vi "RT Driver VI.vi"(7 "Operation":T1, 11 "Device Reference in":T2 format="%.0x") -> (0 "Error Code":i32)   [LabVIEW 2020, in "Ballard MIL-1553 Engine.lvlib"]
uses:
  Ballard MIL-1553 Engine.lvlib
  <vilib>/NI VeriStand/Custom Device API/Custom Device Item Ref.ctl
  <vilib>/NI VeriStand/Custom Device API/Hardware Interface Driver VI Operation.ctl
  RT Driver/Controls/RT StateVariables.ctl
  <vilib>/NI/NIVS Inline Async API/_VS Inline Async API/VS Inline Async API/VS Inline Async API.lvclass
  RT Driver/Controls/Card Parameters.ctl
  Shared/Controls and Global/Initialization Method.ctl
  <vilib>/NI VeriStand/Custom Device API/Data Reference.ctl
  RT Driver/Controls/RT Inline Data_Data Description_Channel.ctl
  RT Driver/Controls/RT Inline Frame Descriptor.ctl
  RT Driver/Controls/RT Inline Frame Descriptor_BC.ctl
  <vilib>/NI VeriStand/Custom Device API/Block Data Reference.ctl
  Shared/EncodeDecode/_typedefs/parameter_config_type.ctl
  Shared/EncodeDecode/_typedefs/parameter_config_type_type.ctl
  Shared/EncodeDecode/_typedefs/parameter_config_encoding_type.ctl
  RT Driver/Controls/RT Inline Frame Descriptor_RT.ctl
  Shared/Controls and Global/RT CWD2.ctl
  Shared/Controls and Global/RT CWD1.ctl
  Shared/Controls and Global/RT messageType.ctl
  <vilib>/NI/NIVS Inline Async API/_VS Inline Async API/VS Inline Async API/VS Inline Async API.lvclass/VS Inline Async API.ctl
  <vilib>/NI/NIVS Inline Async API/_Data Access Engine/Data Access Engine/Data Access Engine.lvclass/Data Access Engine.ctl
  <vilib>/NI/NIVS Inline Async API/_Data Access Engine/Access Type Classes/Write/Write.lvclass/Write.ctl
  <vilib>/NI/NIVS Inline Async API/_Data Access Engine/Access Type Classes/ReadWrite/ReadWrite.lvclass/ReadWrite.ctl
  RT Driver/Controls/Inline_Status_Channels.ctl
  <vilib>/NI/NIVS Inline Async API/_Data Access Engine/Access Type Classes/Read/Read.lvclass/Read.ctl
  <vilib>/NI/NIVS Inline Async API/_Data Access Engine/Data Access Engine/Methods/Data.Engine.Read Data from HW.vi
  <vilib>/NI/NIVS Inline Async API/_VS Inline Async API/Error Handling Process/SubVIs/Error.GetError.vi
  <vilib>/NI/NIVS Inline Async API/_Data Access Engine/Data Access Engine/Methods/Data.Engine.Write Data to HW.vi
  <vilib>/NI/NIVS Inline Async API/_Data Access Engine/Access Type Classes/ReadWrite/ReadWrite.EngineData.vi
  <vilib>/NI/NIVS Inline Async API/_Data Access Engine/Access Type Classes/Write/Write.EngineData.vi
  <vilib>/NI/NIVS Inline Async API/_Data Access Engine/Access Type Classes/Read/Read.EngineData.vi
  <vilib>/NI VeriStand/Custom Device API/NI VeriStand - Get Channel Value by Data Reference.vi
  <vilib>/NI VeriStand/Custom Device API/NI VeriStand - Set Channel Value by Data Reference.vi
  <vilib>/NI VeriStand/Custom Device API/NI VeriStand - Get Channel Values by Block Data Reference.vi
  <vilib>/NI VeriStand/Custom Device API/Global Data Refs.vi
  Shared/Ballard 1553 Shared.lvlib
  <vilib>/NI VeriStand/Custom Device API/Custom Device API.lvlib
panel:
  out "Write time uS":u32
  out "Read time uS":u32
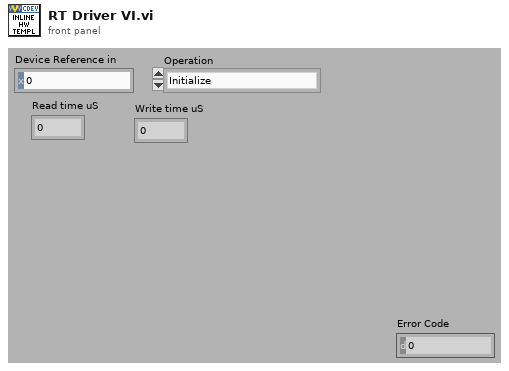
[diagram p1: front panel]
types:
  T1 = typedef "Custom Device API.lvlib/Hardware Interface Driver VI Operation.ctl" = enum16{"Initialize", "Start", "Read Data from HW", "Write Data to HW", "Close"}
  T2 = typedef "Custom Device API.lvlib/Custom Device Item Ref.ctl" = u64
  T3 = typedef "Custom Device API.lvlib/Custom Device Item Info.ctl" = cluster{"Name":string, "Is Channel":bool, "GUID":string, "Is Waveform":bool}
  T4 = typedef "Ballard MIL-1553 Engine.lvlib/RT StateVariables.ctl" = cluster{"Async":refnum<class "VS Inline Async API.lvclass">, "Card Parameters (out)":T5, "Inline Status Channels Refs":T7[], "RT Inline Data_Data Description_Channels":T8[]}
  T5 = typedef "Ballard MIL-1553 Engine.lvlib/Card Parameters.ctl" = cluster{"card number":i32, "core number":i32, "core handle":u64, "core reader handle":u64, "channel handles[]":u64[], "Initialization Method":T6, "PXI slot number":i32}
  T6 = typedef "Ballard 1553 Shared.lvlib/Initialization Method.ctl" = enum16{"PXI Slot Number", "Card Number"}
  T7 = typedef "Custom Device API.lvlib/Data Reference.ctl" = i32
  T8 = typedef "Ballard MIL-1553 Engine.lvlib/RT Inline Data_Data Description_Channel.ctl" = cluster{"hardwareChannel":u16, "First Index for RT2RT Frames":i32, "Frame Drescriptors":T9[]}
  T9 = typedef "Ballard MIL-1553 Engine.lvlib/RT Inline Frame Descriptor.ctl" = cluster{"BC":T10, "RT":T15, "Initialized?":bool, "RT to RT?":bool, "CWD2":T16, "CWD1":T17, "messageType":T18, "Name":string}
  T10 = typedef "Ballard MIL-1553 Engine.lvlib/RT Inline Frame Descriptor_BC.ctl" = cluster{"Timestamp?":bool, "Timestamp Channel Data Reference":T7, "Data Words?":bool, "param block data refs":T11[], "Sw1?":bool, "Sw2?":bool, "Status Channel Refs":T2[], "ParamConfig":T12[], "word_count":u8}
  T11 = typedef "Custom Device API.lvlib/Block Data Reference.ctl" = cluster{"Data Reference":T7, "Offset":u64, "Length":u64}
  T12 = typedef "parameter_config_type.ctl" = cluster{"Name":string, "Type":T13, "Units":string, "Nword":i32, "StartBit":i32, "Size":i32, "LSB_Value":dbl, "Offset":i32, "Encoding":T14}
  T13 = typedef "parameter_config_type_type.ctl" = enum16{"Opaque", "Enum", "Float", "Integer", "Bcd", "Bool"}
  T14 = typedef "parameter_config_encoding_type.ctl" = enum16{"None", "2-complement", "Unsigned"}
  T15 = typedef "Ballard MIL-1553 Engine.lvlib/RT Inline Frame Descriptor_RT.ctl" = cluster{"Timestamp?":bool, "Timestamp Channel Data Reference":T7, "Data Words?":bool, "Words Block Data Refs":T11[], "Status Channel Ref?":bool, "Status Channel Ref":T2, "ParamConfig":T12[], "word_count":u8}
  T16 = typedef "Ballard 1553 Shared.lvlib/RT CWD2.ctl" = cluster{"TA (RT)":i8, "SA":i8, "Words (WC)":i8}
  T17 = typedef "Ballard 1553 Shared.lvlib/RT CWD1.ctl" = cluster{"TA (RT)":i8, "SA":i8, "Mode Code":i8, "Words Count":i8}
  T18 = typedef "Ballard 1553 Shared.lvlib/RT messageType.ctl" = enum16{"BC to RT", "RT to BC", "RT to RT", "MC (Rx)", "MC (Tx)"}
  T19 = typedef "Ballard MIL-1553 Engine.lvlib/Inline_Status_Channels.ctl" = enum16{"Error Code", "Inline Read Time (us)", "Inline Write Time (us)", "Unconfigured Frames Counter", "Monitor - Error Counter", "General Protocol Error Counter", "Wrong Sync Error Counter", "Improper Number of Data Words Error", "Manchester Error Counter", "Parity Error Counter", "Word Error Counter"}
  T20 = typedef "Ballard MIL-1553 Engine.lvlib/RT Async Data.ctl" = cluster{"Map (BC to RT)":T21[], "Raw Values (BC to RT)":T23, "param map (BC to RT)":T25, "Map (RT to ..)":T26[], "Raw Values (RT to ..)":T23, "param map (RT to BC)":T25, "Map (RTs Status)":T27[], "Raw Values (RTs Status)":T23, "Map (Bc Command Channels)":T28[], "MAP (BC Acyclic Messages Trigger)":T29[], "Map (RT Command Channels)":T30[], "Map (MC Rx)":T21[], "Raw Values (MC Rx)":T23, "param map (MC Rx)":T25, "Raw Values (MC Tx)":T23, "Map (MC Tx)":T26[], "param map (MC Tx)":T25}
  T21 = typedef "Ballard MIL-1553 Engine.lvlib/RT Async_Map BC2RT.ctl" = cluster{"Channel Index":i32, "ID":i32, "Channel Data Reference":T7, "Word Index":i32, "Message Handle":u64, "Type":T22, "Word Count":i32, "First Element Index":i32}
  T22 = typedef "Ballard MIL-1553 Engine.lvlib/RT Async_Map_Type.ctl" = enum16{"Word (BC to RT)", "Word (MC (Rx))", "Acyclic Message Trigger", "Word (RT to ..)", "Word (RT to RT)", "Word (MC (Tx))", "RT Status", "BC Commands", "RT Commands"}
  T23 = typedef "Ballard MIL-1553 Engine.lvlib/RT Async_Raw Values.ctl" = cluster{"Association":T24[], "Raw Values Array":u16[]}
  T24 = typedef "Ballard MIL-1553 Engine.lvlib/RT Async_Raw Values to Messages Index_Association.ctl" = cluster{"Message Index":i32, "Raw Value Index":i32}
  T25 = typedef "Ballard MIL-1553 Engine.lvlib/Asynchronous - Parameter map_type.ctl" = cluster{"ParamConfig":T12[], "word_count":u8[], "param_count":u8[]}
  T26 = typedef "Ballard MIL-1553 Engine.lvlib/RT Async_Map RT2BC.ctl" = cluster{"Channel Index":i32, "ID":i32, "Word Data Reference":T7, "First element Index":i32, "rt Transfer Handle":u64, "Type":T22, "Word Count":i32}
  T27 = typedef "Ballard MIL-1553 Engine.lvlib/RT Async_Map RTs Status.ctl" = cluster{"Channel Index":i32, "ID":i32, "rt Transfer Handle":u64, "Type":T22}
  T28 = typedef "Ballard MIL-1553 Engine.lvlib/RT Async_Map BC Command Channels.ctl" = cluster{"Channel Index":i32, "ID":i32, "BC Handle":u64, "Type":T22, "BC Command Channel Ref":T2, "Command Type":enum16{"Start Command", "Stop Command"}}
  T29 = typedef "Ballard MIL-1553 Engine.lvlib/RT Async_Map BC Acyclic Messages Trigger.ctl" = cluster{"Channel Index":i32, "BC Handle":u64, "Type":T22, "Acyclic Message Trigger Channel Ref":T2, "Message Name":string}
  T30 = typedef "Ballard MIL-1553 Engine.lvlib/RT Async_Map RT Command Channels.ctl" = cluster{"Channel Index":i32, "ID":i32, "RT Handle":u64, "Type":T22, "RT Command Channel Ref":T2, "Command Type":enum16{"Start Command", "Stop Command"}}
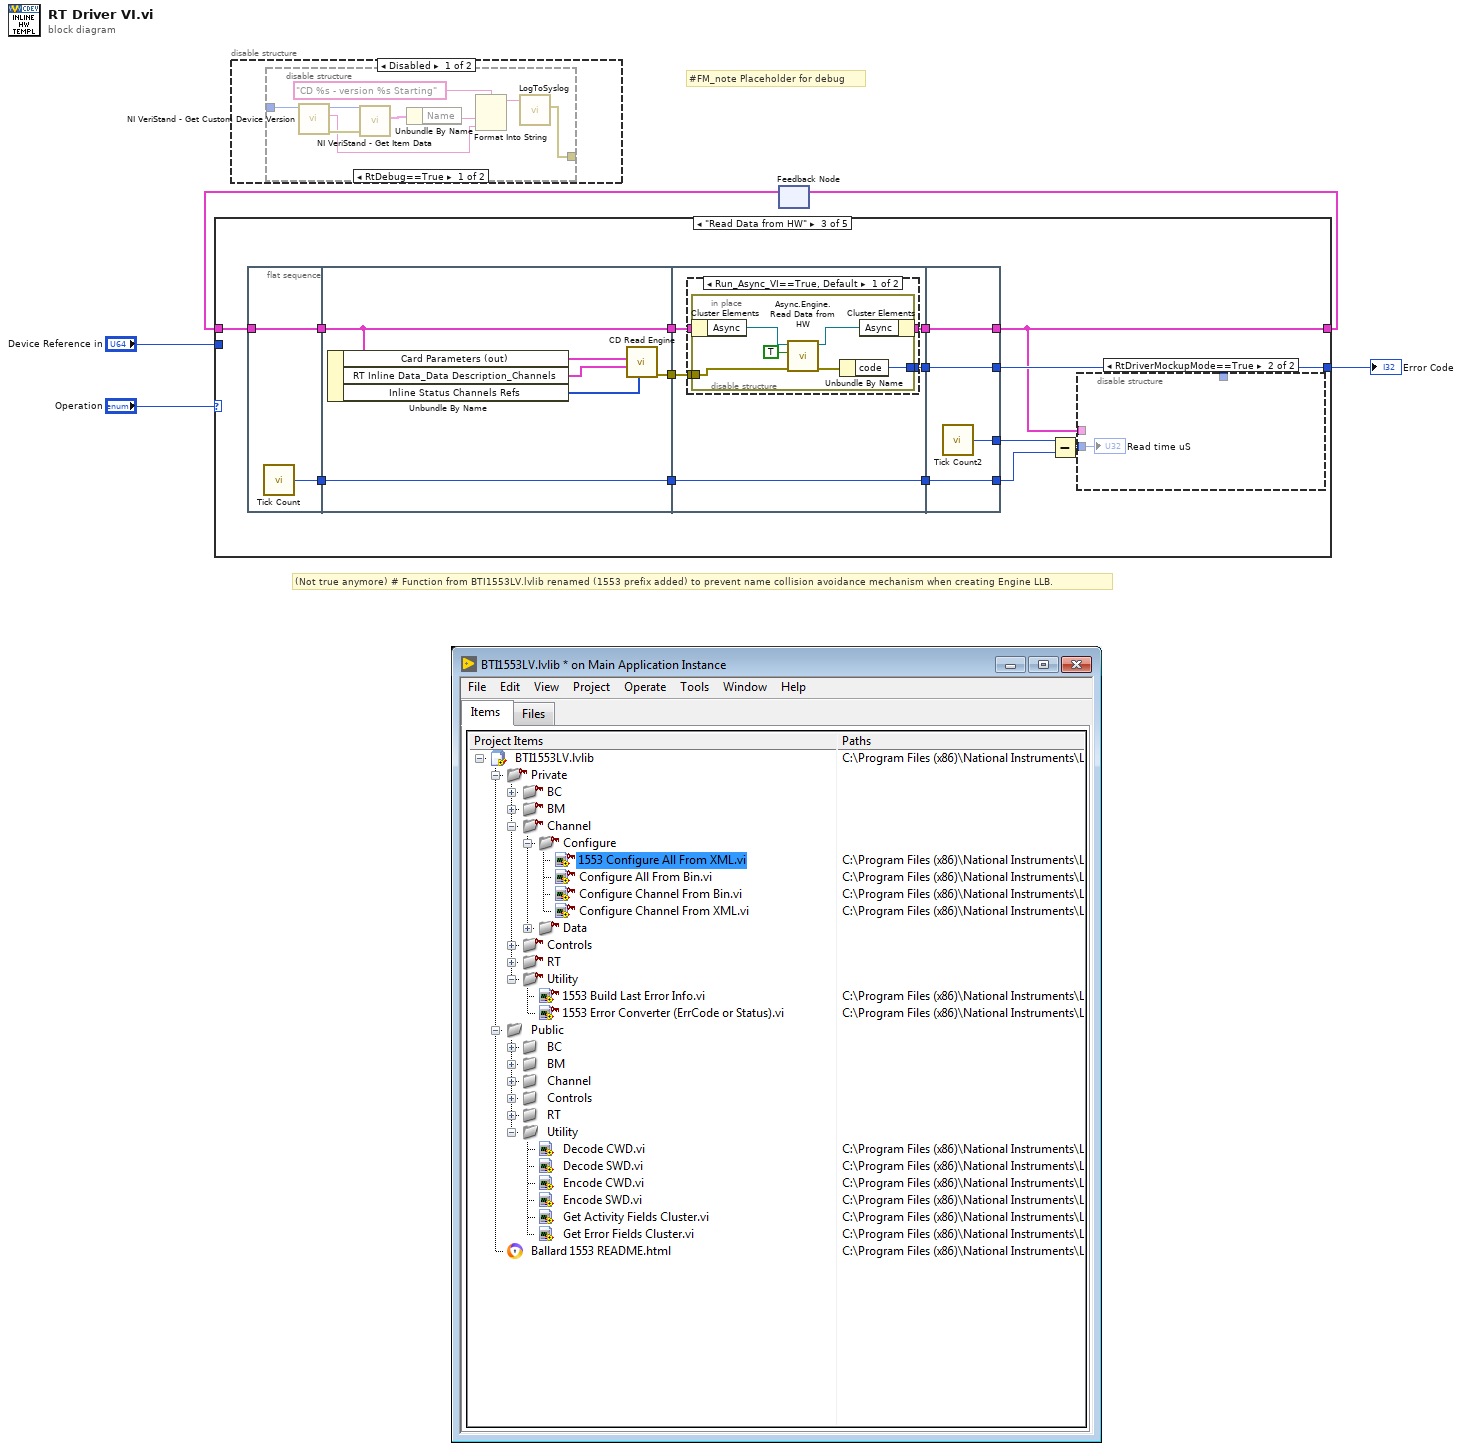
[diagram p0: block diagram]
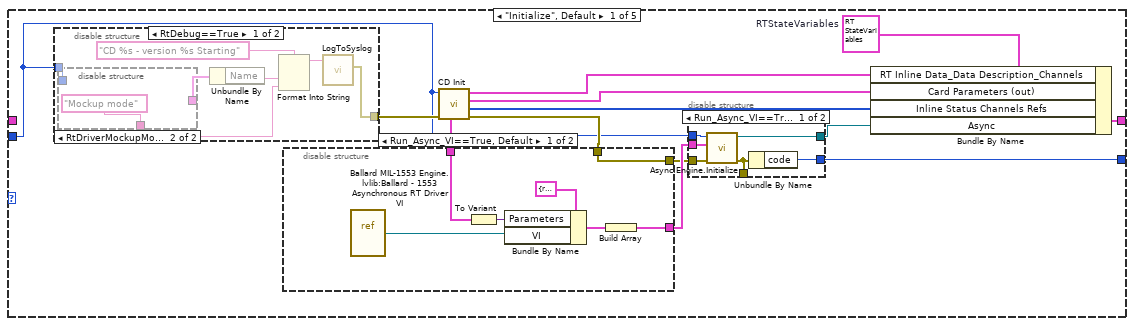
[diagram p4: hidden frame]
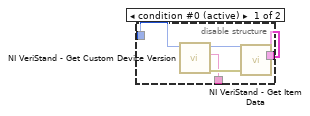
[diagram p5: hidden frame]
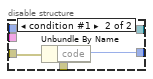
[diagram p8: hidden frame]
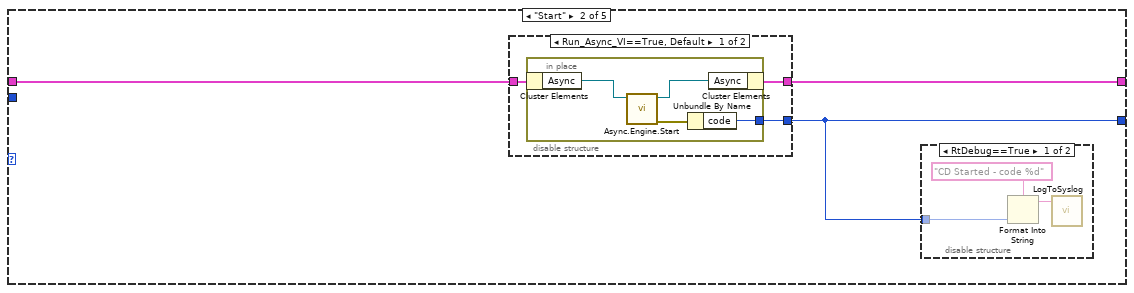
[diagram p9: hidden frame]
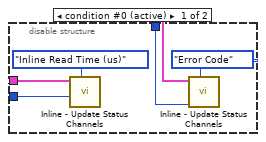
[diagram p12: hidden frame]
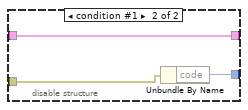
[diagram p13: hidden frame]
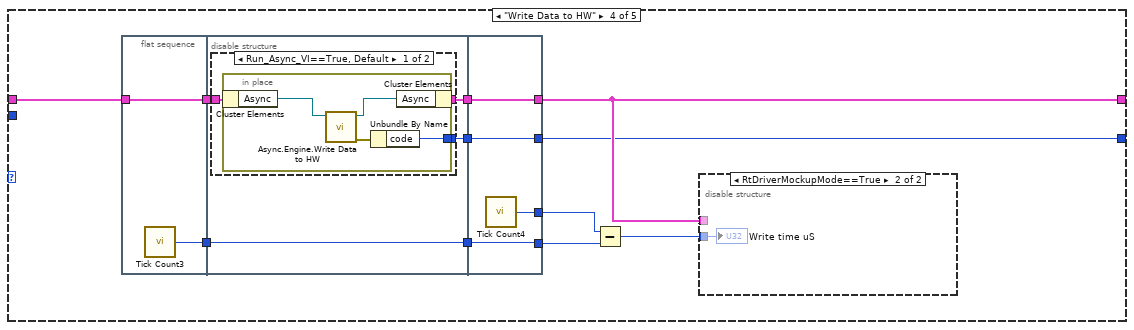
[diagram p14: hidden frame]
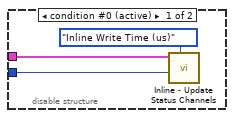
[diagram p15: hidden frame]
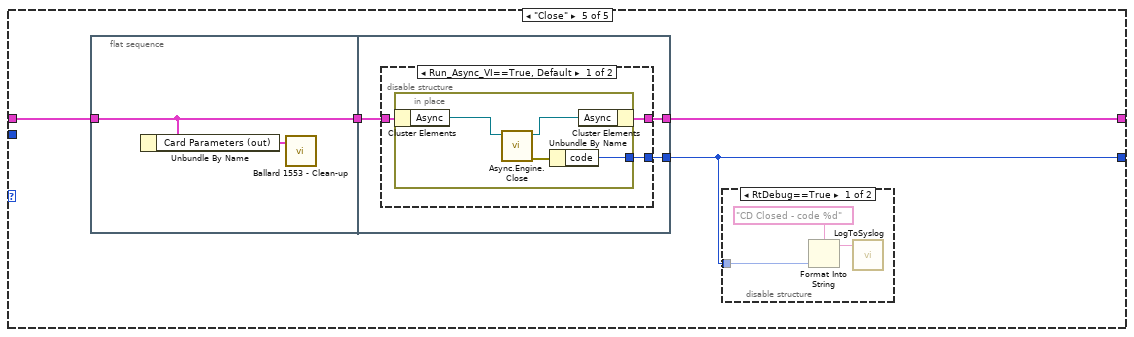
[diagram p17: hidden frame]
diagram:
  # "#FM_note Placeholder for debug"
  # "(Not true anymore) # Function from BTI1553LV.lvlib renamed (1553 prefix added) to prevent name collision avoidance mechanism when creating Engine LLB."
  n1 = disable-structure shown="Disabled" {
    frame Disabled {
      n2 = disable-structure shown="RtDebug==True" {
        disable-tunnel: _ -> [w14 _]
        disable-tunnel: [w8 _] -> _
        frame condition #0 {
          n3 = call <vilib>:"NI VeriStand - Get Custom Device Version.vi"("Device Ref in"=w14) -> ("error out"=w12:errorcluster, "Value"=w6:string, "Device Ref out"=w13:T2)  [unwired: 8 in]
          n4 = call <vilib>:"NI VeriStand - Get Item Data.vi"("error in (no error)"=w12, "Item Ref in"=w13) -> ("Item Info"=w11:T3)  [unwired: 9 out]
          n5 = Unbundle By Name(w11) -> ("Name"=w7:string)
          n6 = Format Into String(format string="CD %s - version %s Starting", w7, w6) -> (resulting string=w10:string)  [unwired: 2 in, 1 out]
          n7 = call "LogToSyslog.vi"("message"=w10) -> ("error out"=w8:errorcluster)  [unwired: 9 in, 1 out]
        }
        frame condition #1 (active) {
        }
      }
    }
    frame Enabled {
    }
  }
  n8 = feedback #1() -> (w4:T4)  [unwired: 1 out]
  n9 = case shown="\"Read Data from HW\"" "Operation" {
    tunnel: [w26 w59 w77 w122 w156] -> w5
    tunnel: w4 -> [_ w58 w84 w131 w157]
    tunnel: "Device Reference in" -> [w15 _ _ _ _]
    tunnel: [w18 w57 w79 w121 w154] -> w1
    frame "Initialize", Default {
      w25 = T4 {"Async"=refnum, "Card Parameters (out)"={"card number"=0, "core number"=0, "core handle"=0, "core reader handle"=0, "channel handles[]"=[], "Initialization Method"=enum."PXI Slot Number", "PXI slot number"=0}, "Inline Status Channels Refs"=[], "RT Inline Data_Data Description_Channels"=[]}  # RTStateVariables
      n10 = disable-structure shown="RtDebug==True" {
        disable-tunnel: w15 -> [w34 _]
        disable-tunnel: [w30 _] -> w16
        frame condition #0 {
          n11 = disable-structure shown="RtDriverMockupMode==True" {
            disable-tunnel: w34 -> [w39 _]
            disable-tunnel: [w36 _] -> w33
            disable-tunnel: [w35 "Mockup mode" ("Value")] -> w28
            frame condition #0 (active) {
              n12 = call <vilib>:"NI VeriStand - Get Custom Device Version.vi"("Device Ref in"=w39) -> ("error out"=w37:errorcluster, "Value"=w35:string, "Device Ref out"=w38:T2)  [unwired: 8 in]
              n13 = call <vilib>:"NI VeriStand - Get Item Data.vi"("error in (no error)"=w37, "Item Ref in"=w38) -> ("Item Info"=w36:T3)  [unwired: 9 out]
            }
            frame condition #1 {
            }
          }
          n14 = Unbundle By Name(w33) -> ("Name"=w29:string)
          n15 = Format Into String(format string="CD %s - version %s Starting", w29, w28) -> (resulting string=w32:string)  [unwired: 2 in, 1 out]
          n16 = call "LogToSyslog.vi"("message"=w32) -> ("error out"=w30:errorcluster)  [unwired: 9 in, 1 out]
        }
        frame condition #1 (active) {
        }
      }
      n17 = call "CD Init.vi"("Error (in)"=w16, "Device Reference"=w15) -> ("Error (out)"=w19:errorcluster, "Inline Status Channels Refs"=w21:T7[], "Card Parameters (out)"=w22:T5, "RT Inline Data_Data Description_Channels"=w23:T8[], "RT Async Data"=w20:T20)  [unwired: 5 in]
      n18 = disable-structure shown="Run_Async_VI==True, Default" {
        disable-tunnel: [w45 _] -> w24
        disable-tunnel: w20 -> [w43 _]
        disable-tunnel: w19 -> [w42 w48]
        disable-tunnel: [w42 w48] -> w17
        frame condition #0 (active) {
          n19 = vi-ref "Ballard MIL-1553 Engine.lvlib:Ballard - 1553 Asynchronous RT Driver VI.vi"() -> (w41:refnum<vi>)
          n20 = To Variant(anything=w43) -> (Variant=w44:variant)
          n21 = Bundle By Name(cluster=cluster{"VI":refnum<vi>, "Parameters":variant} {"VI"=refnum, "Parameters"=variant} ("Process"), "Parameters"=w44, "VI"=w41) -> (w46:cluster{"VI":refnum<vi>, "Parameters":variant})
          n22 = Build Array(w46) -> (w45:cluster{"VI":refnum<vi>, "Parameters":variant}[])
        }
        frame condition #1 {
        }
      }
      n23 = disable-structure shown="Run_Async_VI==True, Default" {
        disable-tunnel: [w54 w55] -> w18
        disable-tunnel: [w53 _] -> w27
        disable-tunnel: w24 -> [w52 _]
        disable-tunnel: w17 -> [w51 w56]
        disable-tunnel: [w50 _] -> _
        disable-tunnel: w15 -> [w49 _]
        frame condition #0 (active) {
          n24 = call <vilib>:"Async.Engine.Initialize.vi"("error in (no error)"=w51, "Processes"=w52, "Custom Device Ref"=w49) -> ("error out"=w50:errorcluster, "Async"=w53:refnum<class "VS Inline Async API.lvclass">)  [unwired: 7 in]
          n25 = Unbundle By Name(w50) -> ("code"=w54:i32)
        }
        frame condition #1 {
          n26 = Unbundle By Name(w56) -> ("code"=w55:i32)
        }
      }
      n27 = Bundle By Name(cluster=w25, "RT Inline Data_Data Description_Channels"=w23, "Card Parameters (out)"=w22, "Inline Status Channels Refs"=w21, "Async"=w27) -> (w26:T4)
    }
    frame "Start" {
      n28 = disable-structure shown="Run_Async_VI==True, Default" {
        disable-tunnel: w58 -> [w65 w70]
        disable-tunnel: [w64 w70] -> w59
        disable-tunnel: [w63 _] -> w57
        frame condition #0 (active) {
          n29 = in-place {
            in-place-border: [w66] -> w63
            n30 = in-place-cluster #2(w65) -> ("Async"=w69:refnum<class "VS Inline Async API.lvclass">)
            n31 = call <vilib>:"Async.Engine.Start.vi"("VS Inline Async API in"=w69) -> ("error out"=w67:errorcluster, "VS Inline Async API out"=w68:refnum<class "VS Inline Async API.lvclass">)  [unwired: 9 in]
            n32 = Unbundle By Name(w67) -> ("code"=w66:i32)
            n33 = in-place-cluster #2("Async"=w68) -> (w64:T4)
          }
        }
        frame condition #1 {
        }
      }
      n34 = disable-structure shown="RtDebug==True" {
        disable-tunnel: w57 -> [w60 _]
        frame condition #0 {
          n35 = Format Into String(format string="CD Started - code %d", w60) -> (resulting string=w62:string)  [unwired: 2 in, 1 out]
          n36 = call "LogToSyslog.vi"("message"=w62) -> ()  [unwired: 9 in, 2 out]
        }
        frame condition #1 (active) {
        }
      }
    }
    frame "Read Data from HW" {
      n37 = flat-sequence {
        tunnel: w84 -> [w92]
        tunnel: [w92] -> w83
        tunnel: [w91] -> w82
        tunnel: [w97] -> w76
        tunnel: [w98] -> w74
        tunnel: w82 -> [w98]
        tunnel: w83 -> [w97]
        tunnel: [w96] -> w71
        tunnel: w76 -> [w102]
        tunnel: [w101] -> w75
        tunnel: w74 -> [w103]
        tunnel: [w103] -> w73
        tunnel: [w99] -> w72
        tunnel: w71 -> [w100]
        tunnel: [w119] -> w77
        tunnel: [w120] -> w79
        tunnel: w75 -> [w119]
        tunnel: [w118] -> w81
        tunnel: w73 -> [w117]
        tunnel: [w117] -> w80
        tunnel: w72 -> [w120]
        frame #0 {
          n38 = call "Tick Count"() -> ("Tick Count(uSec)"=w91:u32)
        }
        frame #1 {
          n39 = Unbundle By Name(w97) -> ("Card Parameters (out)"=w95:T5, "RT Inline Data_Data Description_Channels"=w93:T8[], "Inline Status Channels Refs"=w94:T7[])
          n40 = call "CD Read Engine.vi"("Inline Status Channels Refs"=w94, "RT Inline Data_Data Description_Channels"=w93, "Card Parameters (in)"=w95) -> ("Error (out)"=w96:errorcluster)  [unwired: 7 in]
        }
        frame #2 {
          n41 = disable-structure shown="Run_Async_VI==True, Default" {
            disable-tunnel: [w107 w114] -> w99
            disable-tunnel: w102 -> [w106 w116]
            disable-tunnel: [w105 w116] -> w101
            disable-tunnel: w100 -> [w104 w115]
            frame condition #0 (active) {
              n42 = in-place {
                in-place-border: [w111] -> w107
                in-place-border: w104 -> [w108]
                n43 = in-place-cluster #3(w106) -> ("Async"=w113:refnum<class "VS Inline Async API.lvclass">)
                n44 = call <vilib>:"Async.Engine.Read Data from HW.vi"("error in"=w108, "Report Error to Inline?"=TRUE, "Async in"=w113) -> ("error out"=w110:errorcluster, "Async out"=w112:refnum<class "VS Inline Async API.lvclass">)  [unwired: 7 in]
                n45 = Unbundle By Name(w110) -> ("code"=w111:i32)
                n46 = in-place-cluster #3("Async"=w112) -> (w105:T4)
              }
            }
            frame condition #1 {
              n47 = Unbundle By Name(w115) -> ("code"=w114:i32)
            }
          }
        }
        frame #3 {
          n48 = call "Tick Count2"() -> ("Tick Count(uSec)"=w118:u32)
        }
      }
      n49 = Subtract(x=w81, y=w80) -> (x-y=w78:u32)
      n50 = disable-structure shown="RtDriverMockupMode==True" {
        disable-tunnel: w79 -> [w89 _]
        disable-tunnel: w78 -> [w87 w90]
        disable-tunnel: w77 -> [w86 _]
        frame condition #0 (active) {
          n51 = call "Inline - Update Status Channels.vi"("Status Channel"=Inline_Status_Channels."Inline Read Time (us)", "Time (us)"=w87, "RTStateVariables"=w86) -> ()  [unwired: 9 in]
          n52 = call "Inline - Update Status Channels.vi"("Status Channel"=Inline_Status_Channels."Error Code", "Error Code"=w89, "RTStateVariables"=w86) -> ()  [unwired: 9 in]
        }
        frame condition #1 {
          "Read time uS" <- w90
        }
      }
    }
    frame "Write Data to HW" {
      n53 = flat-sequence {
        tunnel: w131 -> [w137]
        tunnel: [w137] -> w130
        tunnel: [w136] -> w127
        tunnel: w130 -> [w138]
        tunnel: [w141] -> w129
        tunnel: [w140] -> w128
        tunnel: w127 -> [w139]
        tunnel: [w139] -> w126
        tunnel: [w152] -> w122
        tunnel: [w153] -> w121
        tunnel: w129 -> [w153]
        tunnel: w128 -> [w152]
        tunnel: [w151] -> w124
        tunnel: w126 -> [w150]
        tunnel: [w150] -> w125
        frame #0 {
          n54 = call "Tick Count3"() -> ("Tick Count(uSec)"=w136:u32)
        }
        frame #1 {
          n55 = disable-structure shown="Run_Async_VI==True, Default" {
            disable-tunnel: [w144 _] -> w141
            disable-tunnel: w138 -> [w143 w149]
            disable-tunnel: [w142 w149] -> w140
            frame condition #0 (active) {
              n56 = in-place {
                in-place-border: [w148] -> w144
                n57 = in-place-cluster #4(w143) -> ("Async"=w146:refnum<class "VS Inline Async API.lvclass">)
                n58 = call <vilib>:"Async.Engine.Write Data to HW.vi"("VS Inline Async API in"=w146) -> ("error out"=w147:errorcluster, "VS Inline Async API out"=w145:refnum<class "VS Inline Async API.lvclass">)  [unwired: 9 in]
                n59 = Unbundle By Name(w147) -> ("code"=w148:i32)
                n60 = in-place-cluster #4("Async"=w145) -> (w142:T4)
              }
            }
            frame condition #1 {
            }
          }
        }
        frame #2 {
          n61 = call "Tick Count4"() -> ("Tick Count(uSec)"=w151:u32)
        }
      }
      n62 = Subtract(x=w124, y=w125) -> (x-y=w123:u32)
      n63 = disable-structure shown="RtDriverMockupMode==True" {
        disable-tunnel: w123 -> [w134 w135]
        disable-tunnel: w122 -> [w133 _]
        frame condition #0 (active) {
          n64 = call "Inline - Update Status Channels.vi"("Status Channel"=Inline_Status_Channels."Inline Write Time (us)", "Time (us)"=w134, "RTStateVariables"=w133) -> ()  [unwired: 9 in]
        }
        frame condition #1 {
          "Write time uS" <- w135
        }
      }
    }
    frame "Close" {
      n65 = flat-sequence {
        tunnel: w157 -> [w162]
        tunnel: [w162] -> w155
        tunnel: [w164] -> w156
        tunnel: [w163] -> w154
        tunnel: w155 -> [w165]
        frame #0 {
          n66 = Unbundle By Name(w162) -> ("Card Parameters (out)"=w161:T5)
          n67 = call "Ballard 1553 - Clean-up.vi"("Card Parameters"=w161) -> ()  [unwired: 10 in, 1 out]
        }
        frame #1 {
          n68 = disable-structure shown="Run_Async_VI==True, Default" {
            disable-tunnel: w165 -> [w168 w173]
            disable-tunnel: [w167 w173] -> w164
            disable-tunnel: [w166 _] -> w163
            frame condition #0 (active) {
              n69 = in-place {
                in-place-border: [w170] -> w166
                n70 = in-place-cluster #5(w168) -> ("Async"=w172:refnum<class "VS Inline Async API.lvclass">)
                n71 = call <vilib>:"Async.Engine.Close.vi"("Async in"=w172) -> ("error out"=w169:errorcluster, "Async out"=w171:refnum<class "VS Inline Async API.lvclass">)  [unwired: 9 in]
                n72 = Unbundle By Name(w169) -> ("code"=w170:i32)
                n73 = in-place-cluster #5("Async"=w171) -> (w167:T4)
              }
            }
            frame condition #1 {
            }
          }
        }
      }
      n74 = disable-structure shown="RtDebug==True" {
        disable-tunnel: w154 -> [w158 _]
        frame condition #0 {
          n75 = Format Into String(format string="CD Closed - code %d", w158) -> (resulting string=w160:string)  [unwired: 2 in, 1 out]
          n76 = call "LogToSyslog.vi"("message"=w160) -> ()  [unwired: 9 in, 2 out]
        }
        frame condition #1 (active) {
        }
      }
    }
  }
  "Error Code" <- w1
  n77 = feedback-in #1(w5) -> ()
